vi "Force_Idle.vi"(8 "error in (no error)":errorcluster, 10 "Cluster in":T1, 11 "Enum in":T2) -> (0 "error out":errorcluster, 2 "Cluster out":T1, 3 "Enum out":T2)   [LabVIEW 2018]
uses:
  Type_Def/Type_Def ControlState.ctl
  Type_Def/Type_Def Actuator Controls.ctl
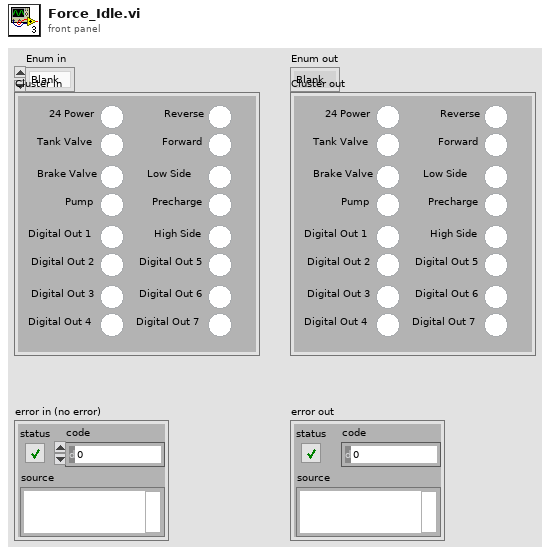
[diagram p1: front panel]
types:
  T1 = typedef "Type_Def Actuator Controls.ctl" = cluster{"Reverse ":bool, "Forward":bool, "Low Side":bool, "Precharge":bool, "High Side":bool, "Digital Out 5":bool, "Digital Out 6":bool, "Digital Out 7 ":bool, "24 Power":bool, "Tank Valve ":bool, "Brake Valve":bool, "Pump":bool, "Digital Out 1 ":bool, "Digital Out 2":bool, "Digital Out 3":bool, "Digital Out 4 ":bool}
  T2 = typedef "Type_Def ControlState.ctl" = enum16{"Blank", "Systems Check", "Idle", "Ready", "Pushing", "CrawlingPrecharge", "Braking", "Fault", "Boot Up", "Unpowered", "Crawling", "Shutdown", "Service Push", "Service Wait", "Vent", "Precharge", "Cooldown"}
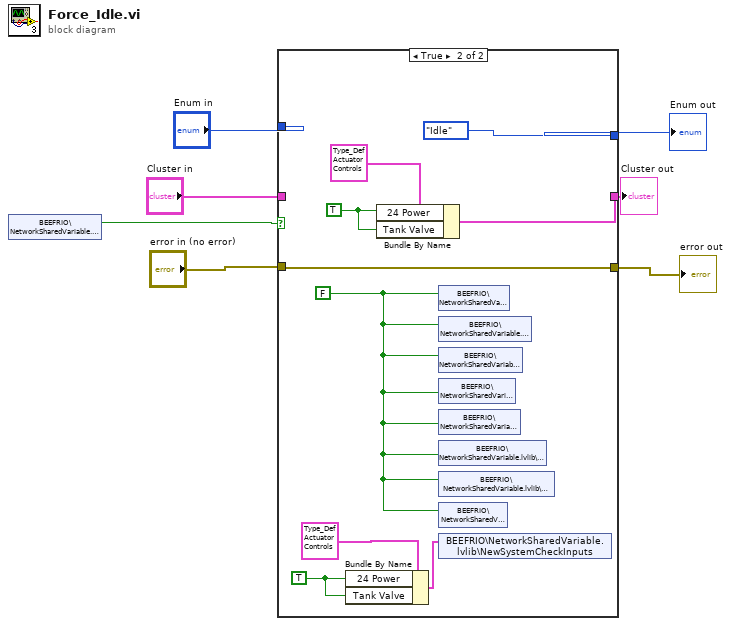
[diagram p0: block diagram]
diagram:
  n1 = shared-variable "BEEFRIO\\NetworkSharedVariable.lvlib\\ForceIdle"() -> (w1:bool)  [unwired: 1 in, 1 out]
  n2 = case shown="True" w1 {
    tunnel: [w10 w15] -> w7
    tunnel: "error in (no error)" -> [w10 w15]
    tunnel: [w9 w17] -> w5
    tunnel: "Cluster in" -> [w9 _]
    tunnel: [w8 Type_Def_ControlState."Idle" ("Enum in")] -> w3
    tunnel: "Enum in" -> [w8 _]
    frame False {
    }
    frame True {
      w11 = TRUE ("24 Power")
      w14 = FALSE
      w16 = TRUE
      n3 = Bundle By Name(cluster=T1 {"Reverse "=FALSE, "Forward"=FALSE, "Low Side"=FALSE, "Precharge"=FALSE, "High Side"=FALSE, "Digital Out 5"=FALSE, "Digital Out 6"=FALSE, "Digital Out 7 "=FALSE, "24 Power"=FALSE, "Tank Valve "=FALSE, "Brake Valve"=FALSE, "Pump"=FALSE, "Digital Out 1 "=FALSE, "Digital Out 2"=FALSE, "Digital Out 3"=FALSE, "Digital Out 4 "=FALSE} ("Cluster in 2"), "24 Power"=w11, "Tank Valve"=w11) -> (w12:T1)
      n4 = Bundle By Name(cluster=T1 {"Reverse "=FALSE, "Forward"=FALSE, "Low Side"=FALSE, "Precharge"=FALSE, "High Side"=FALSE, "Digital Out 5"=FALSE, "Digital Out 6"=FALSE, "Digital Out 7 "=FALSE, "24 Power"=FALSE, "Tank Valve "=FALSE, "Brake Valve"=FALSE, "Pump"=FALSE, "Digital Out 1 "=FALSE, "Digital Out 2"=FALSE, "Digital Out 3"=FALSE, "Digital Out 4 "=FALSE} ("Cluster in"), "24 Power"=w16, "Tank Valve"=w16) -> (w17:T1)
      n5 = shared-variable "BEEFRIO\\NetworkSharedVariable.lvlib\\Fault"(w14) -> ()  [unwired: 1 in, 1 out]
      n6 = shared-variable "BEEFRIO\\NetworkSharedVariable.lvlib\\ForceIdle"(w14) -> ()  [unwired: 1 in, 1 out]
      n7 = shared-variable "BEEFRIO\\NetworkSharedVariable.lvlib\\Launch"(w14) -> ()  [unwired: 1 in, 1 out]
      n8 = shared-variable "BEEFRIO\\NetworkSharedVariable.lvlib\\Ready"(w14) -> ()  [unwired: 1 in, 1 out]
      n9 = shared-variable "BEEFRIO\\NetworkSharedVariable.lvlib\\Service"(w14) -> ()  [unwired: 1 in, 1 out]
      n10 = shared-variable "BEEFRIO\\NetworkSharedVariable.lvlib\\ServicePush"(w14) -> ()  [unwired: 1 in, 1 out]
      n11 = shared-variable "BEEFRIO\\NetworkSharedVariable.lvlib\\SystemCheck"(w14) -> ()  [unwired: 1 in, 1 out]
      n12 = shared-variable "BEEFRIO\\NetworkSharedVariable.lvlib\\Vent"(w14) -> ()  [unwired: 1 in, 1 out]
      n13 = shared-variable "BEEFRIO\\NetworkSharedVariable.lvlib\\NewSystemCheckInputs"(w12) -> ()  [unwired: 1 in, 1 out]
    }
  }
  "Enum out" <- w3
  "error out" <- w7
  "Cluster out" <- w5
